vi "Get Scope Mode.vi"(8 "error in (no error)":errorcluster, 11 "VISA resource name":refnum<visa-resource-name>) -> (0 "error out":errorcluster, 2 "Scope Mode":i32, 3 "VISA resource name out":refnum<visa-resource-name>)   [LabVIEW 2014, in "Fluke 5XXX Series Multicalibrators.lvlib"]
doc: "This VI returns the oscilloscope’s current mode of operation.\n\nNote:\n\nThis VI is available only for instrument models 5500A and 5520A with oscilloscope option SC300 (SC600 or SC1100)."
uses:
  Fluke 5XXX Series Multicalibrators.lvlib
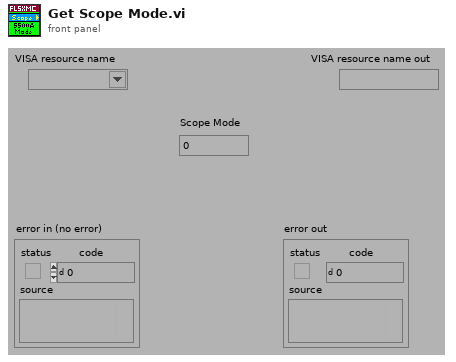
[diagram p1: front panel]
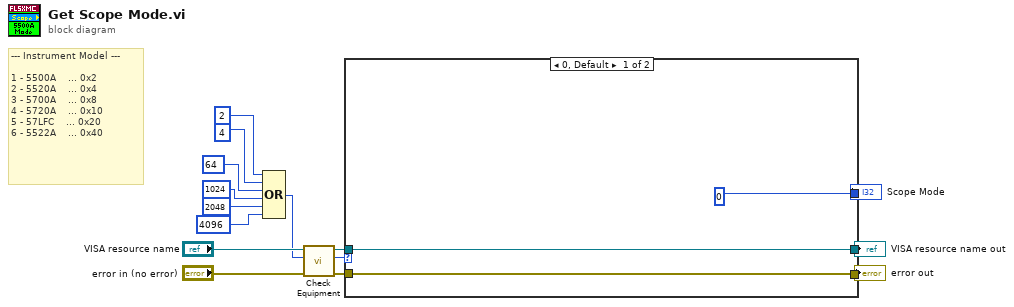
[diagram p0: block diagram]
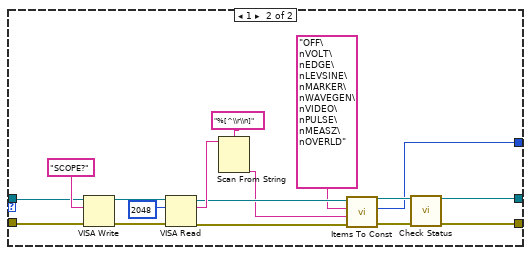
[diagram p2: hidden frame]
diagram:
  # "--- Instrument Model ---\n\n1 - 5500A    ... 0x2\n2 - 5520A    ... 0x4\n3 - 5700A    ... 0x8\n4 - 5720A    ... 0x10\n5 - 57LFC    ... 0x20\n6 - 5522A    ... 0x40"
  n1 = Compound Arithmetic op=OR(2 ("Numeric"), 4 ("Numeric"), 64 ("Numeric"), 1024 ("Numeric"), 2048 ("Numeric"), 4096 ("Numeric")) -> (w3:i32)
  n2 = call "Check Equipment.vi"("error in (no error)"="error in (no error)", "Bit Mask"=w3, "VISA resource name"="VISA resource name") -> ("error out"=w15:errorcluster, "Present?"=w14:u32, "VISA resource name out"=w13:refnum<visa-resource-name>)  [unwired: 6 in]
  n3 = case shown="0, Default" w14 {
    tunnel: [w18 w29] -> w10
    tunnel: [w17 w28] -> w9
    tunnel: w15 -> [w18 w31]
    tunnel: w13 -> [w17 w30]
    tunnel: [0 w20] -> w8
    frame 0, Default {
    }
    frame 1 {
      n4 = VISA Write(VISA resource name=w30, write buffer="SCOPE?", error in (no error)=w31) -> (VISA resource name out=w34:refnum<visa-resource-name>, error out=w33:errorcluster)  [unwired: 1 out]
      n5 = VISA Read(VISA resource name=w34, byte count=u32 2048 ("byte count (0)"), error in (no error)=w33) -> (VISA resource name out=w22:refnum<visa-resource-name>, read buffer=w26:string, error out=w23:errorcluster)  [unwired: 1 out]
      n6 = Scan From String(format string="%[^\\r\\n]", input string=w26) -> (output 1=w21:string)  [unwired: 3 in, 3 out]
      n7 = call "Items To Const.vi"("error in (no error)"=w23, "String Item"=w21, "Multi-Line String"="OFF\nVOLT\nEDGE\nLEVSINE\nMARKER\nWAVEGEN\nVIDEO\nPULSE\nMEASZ\nOVERLD", "VISA resource name"=w22) -> ("error out"=w24:errorcluster, "Index"=w20:i32, "VISA resource name out"=w25:refnum<visa-resource-name>)  [unwired: 5 in]
      n8 = call "Check Status.vi"("VISA resource name"=w25, "error in (no error)"=w24) -> ("VISA resource name out"=w28:refnum<visa-resource-name>, "error out"=w29:errorcluster)  [unwired: 12 in]
    }
  }
  "Scope Mode" <- w8
  "VISA resource name out" <- w9
  "error out" <- w10
